vi "cRIO_v3.vi"() -> ()   [LabVIEW 2015]
uses:
  <vilib>/FPGAPlugInAG/cRIO-9113/niLvFpga_Open_cRIO-9113.vi
  <vilib>/rvi/interface/common/dynamic/niFpgaDynamicAddResources.vi
  <vilib>/Utility/error.llb/Error Cluster From Error Code.vi
  <vilib>/FPGAPlugInAG/Dynamic/niLvFpga_Run_Dynamic.vi
  <vilib>/rvi/interface/common/niFpgaWaitOnOcc.vi
  <vilib>/rvi/errors/niLvFpgaAdjustHostInterfaceError.vi
  <vilib>/FPGAPlugInAG/Dynamic/niLvFpga_Close_Dynamic.vi
  <vilib>/rvi/interface/nirviOpenFPGA/nirviOpenFPGA.xnode
  FPGA Bitfiles/DW40ticks_FPGATarget_Fpgav5_W8FHHtuBRbs.lvbitx
  <vilib>/rvi/interface/nirviMethod/nirviMethod.xnode
  <vilib>/rvi/interface/nirviReadWriteControl/nirviReadWriteControl.xnode
  <vilib>/rvi/interface/nirviCloseFPGA/nirviCloseFPGA.xnode
  <vilib>/rvi/errors/niLvFpgaMergeErrorWithErrorCode.vi
  <vilib>/FPGAPlugInAG/Dynamic/niLvFpga_ReadFifo_Dynamic.vi
  <vilib>/rvi/interface/Simulation/niFpgaSimulationCallBeginRW.vi
  NiFpgaLv.dll
  <vilib>/FPGAPlugInAG/Dynamic/niLvFpga_StartFifo_Dynamic.vi
  <vilib>/FPGAPlugInAG/Dynamic/niLvFpga_ConfigureFifo_Dynamic.vi
panel:
  out "Waveform Graph":u32[](graph)
  out "x-y 3":u32
  in  "Stop fpga":bool
  out "error out":errorcluster
  out "Actual Depth of FIFO":u32
  out "Initial write Elements Remaining":u32
  in  "stop":bool
  out "Timed Out?":bool
  out "Number of times timed out":u8
  out "backlog (Elements remaing on the write)":u32
  in  "Data write ON/OFF":bool
  out "Time(ms) for a loop":u32
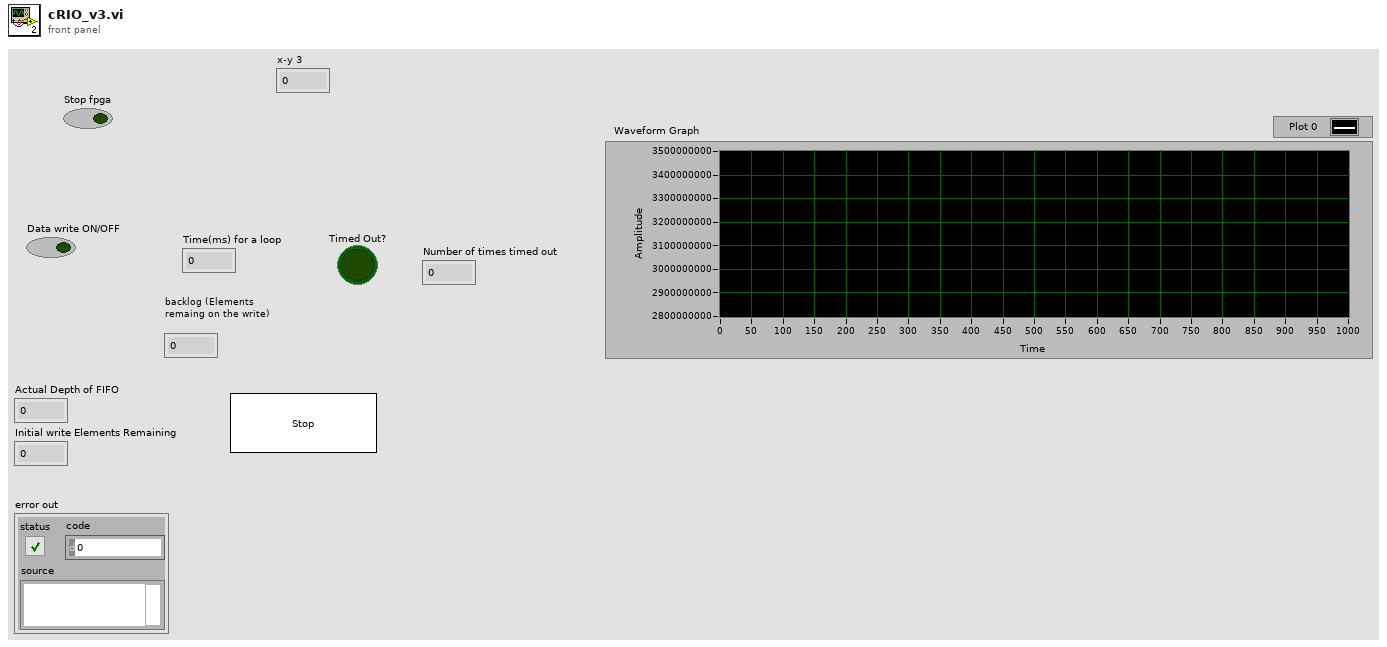
[diagram p1: front panel]
types:
  T1 = enum16{"open", "open or create", "create or replace", "create", "open (read-only)"}
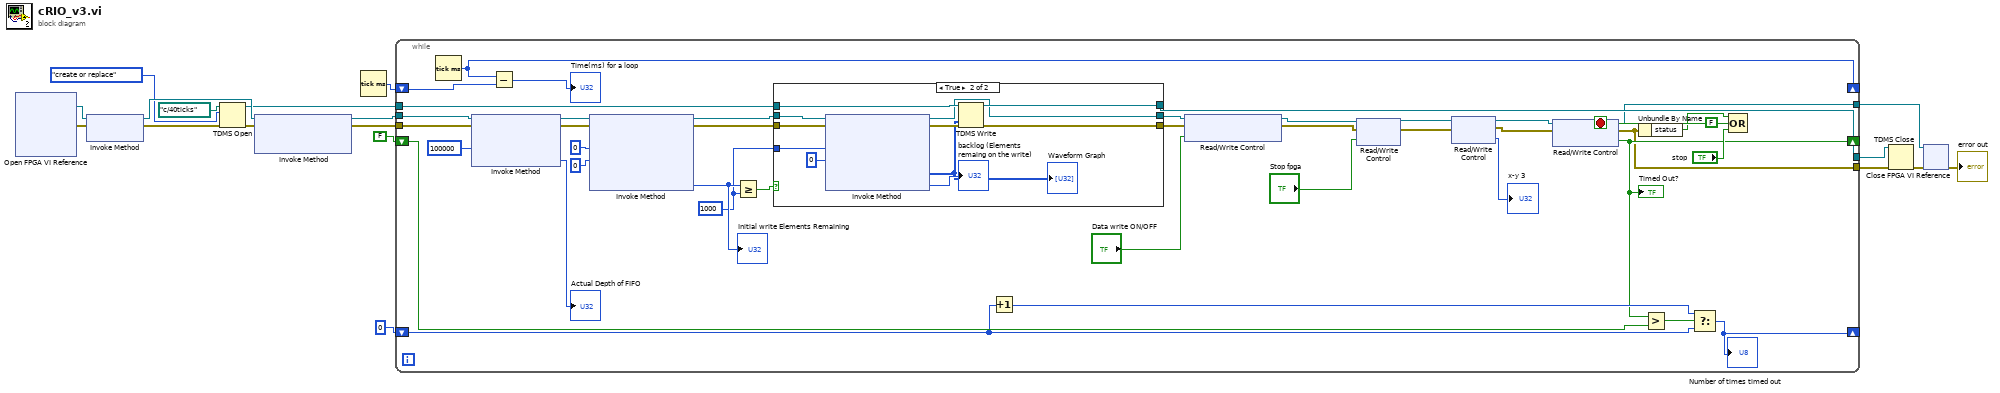
[diagram p0: block diagram]
diagram:
  n1 = xnode "Open FPGA VI Reference"() -> ("FPGA VI Reference Out"=w1:refnum<k20>, "error out"=w2:errorcluster)  [unwired: 2 in]
  n2 = xnode "Invoke Method"("FPGA VI Reference In"=w1, "error in"=w2) -> ("FPGA VI Reference Out"=w17:refnum<k20>, "error out"=w18:errorcluster)
  n3 = TDMS Open(8:w18, 10:T1."create or replace" ("operation (0:open)"), 11:path "c:/40ticks" ("file path")) -> (0:w16:errorcluster, 3:w11:refnum<k34>)  [unwired: 4 in]
  n4 = xnode "Invoke Method"("FPGA VI Reference In"=w17, "error in"=w16) -> ("FPGA VI Reference Out"=w15:refnum<k20>, "error out"=w14:errorcluster)  [unwired: 1 in]
  n5 = Tick Count (ms)() -> (millisecond timer value=w3:u32)
  n6 = while {
    tunnel: w15 -> [w59]
    tunnel: w14 -> [w58]
    tunnel: w11 -> [w50]
    tunnel: [w48] -> w9
    shift-right: [w33] -> _
    shift-left: FALSE ("Timed Out?") -> [w46]
    shift-right: [w42] -> _
    shift-left: u8 0 -> [w44]
    tunnel: [w28] -> w5
    tunnel: [w27] -> w4
    shift-right: [w31] -> _
    shift-left: w3 -> [w32]
    stop <- w47 stop-if-true
    w37 = u32 1000 ("y")
    n7 = Tick Count (ms)() -> (millisecond timer value=w31:u32)
    n8 = xnode "Invoke Method"("FPGA VI Reference In"=w59, "error in"=w58, "Requested Depth"=u32 100000) -> ("FPGA VI Reference Out"=w55:refnum<k20>, "error out"=w54:errorcluster, "Actual Depth"=→"Actual Depth of FIFO":u32)
    n9 = Subtract(x=w31, y=w32) -> (x-y=→"Time(ms) for a loop":u32)
    n10 = xnode "Invoke Method"("FPGA VI Reference In"=w55, "error in"=w54, "Number of Elements"=u32 0, "Timeout (ms)"=0) -> ("FPGA VI Reference Out"=w38:refnum<k20>, "error out"=w51:errorcluster, "Elements Remaining"=w39:u32)  [unwired: 1 out]
    "Initial write Elements Remaining" <- w39
    n11 = Greater Or Equal?(x=w39, y=w37) -> (x >= y?=w40:bool)
    n12 = case shown="True" w40 {
      tunnel: w51 -> [w60 w69]
      tunnel: w50 -> [w62 w73]
      tunnel: [w60 w72] -> w35
      tunnel: [w62 w71] -> w48
      tunnel: w38 -> [w61 w70]
      tunnel: [w61 w68] -> w36
      tunnel: w37 -> [_ w66]
      frame False {
      }
      frame True {
        n13 = xnode "Invoke Method"("FPGA VI Reference In"=w70, "error in"=w69, "Number of Elements"=w66, "Timeout (ms)"=0) -> ("FPGA VI Reference Out"=w68:refnum<k20>, "error out"=w67:errorcluster, "Data"=w63:u32[], "Elements Remaining"=→"backlog (Elements remaing on the write)":u32)
        "Waveform Graph" <- w63
        n14 = TDMS Write(0:w73, 9:w63, 11:w67) -> (4:w71:refnum<k34>, 15:w72:errorcluster)  [unwired: 3 in, 2 out]
      }
    }
    n15 = Increment(x=w44) -> (x+1=w43:u8)
    n16 = xnode "Read/Write Control"("FPGA VI Reference In"=w36, "error in"=w35, "Data write ON/OFF"="Data write ON/OFF") -> ("FPGA VI Reference Out"=w26:refnum<k20>, "error out"=w25:errorcluster)
    n17 = xnode "Read/Write Control"("FPGA VI Reference In"=w26, "error in"=w25, "stop"="Stop fpga") -> ("FPGA VI Reference Out"=w23:refnum<k20>, "error out"=w22:errorcluster)
    n18 = xnode "Read/Write Control"("FPGA VI Reference In"=w23, "error in"=w22) -> ("FPGA VI Reference Out"=w20:refnum<k20>, "error out"=w21:errorcluster, "x-y 3"=→"x-y 3":u32)
    n19 = xnode "Read/Write Control"("FPGA VI Reference In"=w20, "error in"=w21) -> ("FPGA VI Reference Out"=w28:refnum<k20>, "error out"=w27:errorcluster, "Timed Out?"=w33:bool)
    "Timed Out?" <- w33
    n20 = Unbundle By Name(w27) -> ("status"=w41:bool)
    n21 = Greater?(x=w33, y=w46) -> (0:w45:bool)
    n22 = Select(t=w43, s=w45, f=w44) -> (s? t:f=w42:u8)
    "Number of times timed out" <- w42
    n23 = Compound Arithmetic op=OR(w41, FALSE ("value"), "stop") -> (w47:bool)
  }
  n24 = TDMS Close(8:w4, 11:w9) -> (0:w10:errorcluster)  [unwired: 1 out]
  n25 = xnode "Close FPGA VI Reference"("FPGA VI Reference In"=w5, "error in"=w10) -> ("error out"=→"error out":errorcluster)
